vi "vi server fun.vi"() -> ()   [LabVIEW 2021]
uses:
  <vilib>/Utility/LVLibp/NI_PackedLibraryUtility.lvlib
panel:
  out "error out":errorcluster
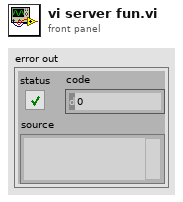
[diagram p1: front panel]
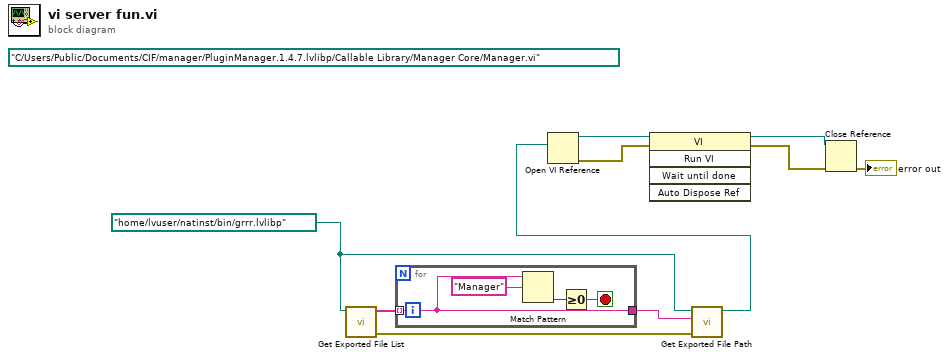
[diagram p0: block diagram]
diagram:
  w2 = path "/home/lvuser/natinst/bin/grrr.lvlibp" ("vi path")
  (unwired) path "C:/Users/Public/Documents/CIF/manager/PluginManager.1.4.7.lvlibp/Callable Library/Manager Core/Manager.vi" ("vi path")
  n1 = call <vilib>:"Get Exported File List.vi"("packed library path"=w2) -> ("error out"=w3:errorcluster, "qualified names"=w5:string[])  [unwired: 8 in, 1 out]
  n2 = for {
    tunnel: w5 -> [w11] mode=indexing
    tunnel: [w11] -> w4
    stop <- w13 stop-if-true
    n3 = Match Pattern(string=w11, regular expression="Manager") -> (offset past match=w14:i32)  [unwired: 1 in, 3 out]
    n4 = Greater Or Equal To 0?(x=w14) -> (x >= 0?=w13:bool)
  }
  n5 = call <vilib>:"Get Exported File Path.vi"("error in (no error)"=w3, "qualified name"=w4, "packed library path"=w2) -> ("path"=w1:path)  [unwired: 7 in, 1 out]
  n6 = Open VI Reference(vi path=w1) -> (vi reference=w10:refnum<vi>, error out=w7:errorcluster)  [unwired: 5 in]
  n7 = invoke class="VI" method="Run VI"(reference=w10, error in=w7) -> (reference out=w9:refnum<vi>, error out=w8:errorcluster)  [unwired: 3 in, 3 out]
  n8 = Close Reference(reference=w9, error in (no error)=w8) -> (error out=→"error out":errorcluster)
